vi "Lock to GPS.vi"(0 "niUsrpRio Session":T1={"FPGA Interface"=refnum, "RIO Interface Number"=0, "Data Clock Rate"=0, "FPGA Data Clock Rate"=0, "Global Settings Register Bus"=refnum, "Radio 0 Settings Register Bus"=refnum, "Radio 1 Settings Register Bus"=refnum, "Radio Settings Bus Semaphore"=refnum, "DB Queues"=[], "Characterization Data Valid?"=FALSE, "EEPROM Header"={"Checksum"=0, "Product Code"=0, "Hardware Current Version"=0, "Hardware Oldest Compatible Version"=0, "EEPROM Map Current Version"=0, "EEPROM Map Oldest Compatible Version"=0, "User Password"="", "Pointer to Factory Header"=0, "Pointer to User Header"=0, "Recommended Interval"=0, "Number of Reserved Bytes"=9, "Number of Daughterboards"=0, "Daughterboard IDs"=[], "Daughterboard Serial Numbers"=[]}, "Device Data Header"={"Checksum"=0, "Number of Channels"=0, "Number of Gain Settings"=[], "Pointer to Characterization Data"=[], "Number of Reserved Bytes"=27, "Number of Frequencies"=[]}, "EEPROM Characterization Header"={"Checksum"=0, "Date"=timestamp(0 s since 1904-01-01), "Temperature"=0.0, "Misc. Info"="", "Pointer to Device Data Header"=0, "Number of Reserved Bytes"=28}, "Characterization Data"=[], "FPGA Current Version"=0, "FPGA Oldest Compatible Version"=0, "Fixed Logic Current Version"=0, "Fixed Logic Oldest Compatible Version"=0, "FPGA Radio Settings Bus Current Version"=0, "FPGA Radio Settings Bus Oldest Compatible Version"=0, "FPGA Board Config Current Version"=0, "FPGA Board Config Oldest Compatible Version"=0, "Daughterboard Clock Rate"=0, "daughterboard configuration session handles"=[]} {"Daughterboard Clock Rate" format="%#.3pHz"; "FPGA Data Clock Rate" format="%#.3pHz"; "Data Clock Rate" format="%#.3pHz"; "Characterization Data"."Frequencies [Hz]" format="%#_6p"; "EEPROM Characterization Header"."Pointer to Device Data Header" format="%x"; "EEPROM Characterization Header"."Checksum" format="%x"; "Device Data Header"."Pointer to Characterization Data" format="%x"; "Device Data Header"."Checksum" format="%x"; "EEPROM Header"."Pointer to User Header" format="%x"; "EEPROM Header"."Pointer to Factory Header" format="%x"; "EEPROM Header"."Product Code" format="%x"; "EEPROM Header"."Checksum" format="%x"}, 1 "scope":string, 11 "error in":errorcluster) -> (4 "niUsrpRio Session (out)":T1={"FPGA Interface"=refnum, "RIO Interface Number"=0, "Data Clock Rate"=0, "FPGA Data Clock Rate"=0, "Global Settings Register Bus"=refnum, "Radio 0 Settings Register Bus"=refnum, "Radio 1 Settings Register Bus"=refnum, "Radio Settings Bus Semaphore"=refnum, "DB Queues"=[], "Characterization Data Valid?"=FALSE, "EEPROM Header"={"Checksum"=0, "Product Code"=0, "Hardware Current Version"=0, "Hardware Oldest Compatible Version"=0, "EEPROM Map Current Version"=0, "EEPROM Map Oldest Compatible Version"=0, "User Password"="", "Pointer to Factory Header"=0, "Pointer to User Header"=0, "Recommended Interval"=0, "Number of Reserved Bytes"=9, "Number of Daughterboards"=0, "Daughterboard IDs"=[], "Daughterboard Serial Numbers"=[]}, "Device Data Header"={"Checksum"=0, "Number of Channels"=0, "Number of Gain Settings"=[], "Pointer to Characterization Data"=[], "Number of Reserved Bytes"=27, "Number of Frequencies"=[]}, "EEPROM Characterization Header"={"Checksum"=0, "Date"=timestamp(0 s since 1904-01-01), "Temperature"=0.0, "Misc. Info"="", "Pointer to Device Data Header"=0, "Number of Reserved Bytes"=28}, "Characterization Data"=[], "FPGA Current Version"=0, "FPGA Oldest Compatible Version"=0, "Fixed Logic Current Version"=0, "Fixed Logic Oldest Compatible Version"=0, "FPGA Radio Settings Bus Current Version"=0, "FPGA Radio Settings Bus Oldest Compatible Version"=0, "FPGA Board Config Current Version"=0, "FPGA Board Config Oldest Compatible Version"=0, "Daughterboard Clock Rate"=0, "daughterboard configuration session handles"=[]} {"Daughterboard Clock Rate" format="%#.3pHz"; "FPGA Data Clock Rate" format="%#.3pHz"; "Data Clock Rate" format="%#.3pHz"; "Characterization Data"."Frequencies [Hz]" format="%#_6p"; "EEPROM Characterization Header"."Pointer to Device Data Header" format="%x"; "EEPROM Characterization Header"."Checksum" format="%x"; "Device Data Header"."Pointer to Characterization Data" format="%x"; "Device Data Header"."Checksum" format="%x"; "EEPROM Header"."Pointer to User Header" format="%x"; "EEPROM Header"."Pointer to Factory Header" format="%x"; "EEPROM Header"."Product Code" format="%x"; "EEPROM Header"."Checksum" format="%x"}, 15 "error out":errorcluster)   [LabVIEW 2020]
doc: "Locks to GPS. This VI blocks until the device locks to a GPS signal.\n\nThis VI will take between 10 seconds and 10 minutes to execute. The GPSDO requires 10 seconds at power on before polling for its lock status, and the GPSDO may take up to 10 minutes to acquire a GPS lock."
uses:
  <instrlib>/niUsrpRio/Config/v1/Host/Public/niUsrpRio Session.ctl
  <instrlib>/_niInstr/Register Bus/v0/Host/Public/Register Bus Session.ctl
  <instrlib>/_niInstr/Register Bus/v0/Host/Private/Session Data.ctl
  <instrlib>/niUsrpRio/Config/v1/Host/Private/DB Queue Reference.ctl
  <instrlib>/niUsrpRio/Config/v1/Host/Private/Daughterboard Data.ctl
  <instrlib>/niUsrpRio/Config/v1/Host/Private/ATR state data.ctl
  <instrlib>/niUsrpRio/Config/v1/Host/Private/Antenna Configuration.ctl
  <instrlib>/niUsrpRio/Config/v1/Host/Private/CPLD Power Mode.ctl
  <instrlib>/niUsrpRio/Config/v1/Host/Public/EEPROM Header.ctl
  <instrlib>/niUsrpRio/Config/v1/Host/Public/EEPROM Device Data Header.ctl
  <instrlib>/niUsrpRio/Config/v1/Host/Public/EEPROM Characterization Header.ctl
  <instrlib>/niUsrpRio/Config/v1/Host/Public/Characterization Data.ctl
  <instrlib>/niUsrpRio/Config/v1/Host/Public/IQ Imbalance.ctl
  <instrlib>/niUsrpRio/Config/v1/Host/Public/What to Wait for.ctl
  <instrlib>/niUsrpRio/Config/v1/Host/niUsrpRio Config v1 Host.lvlib
  <instrlib>/_niInstr/Register Bus/v0/Host/niInstr Register Bus v0 Host.lvlib
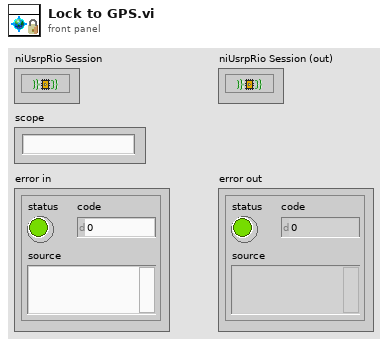
[diagram p1: front panel]
types:
  T1 = typedef "niUsrpRio Config v1 Host.lvlib/niUsrpRio Session.ctl" = cluster{"FPGA Interface":refnum<k20>, "RIO Interface Number":u32, "Data Clock Rate":u32, "FPGA Data Clock Rate":u32, "Global Settings Register Bus":T2, "Radio 0 Settings Register Bus":T2, "Radio 1 Settings Register Bus":T2, "Radio Settings Bus Semaphore":T3, "DB Queues":T4[], "Characterization Data Valid?":bool, "EEPROM Header":T5, "Device Data Header":T6, "EEPROM Characterization Header":T7, "Characterization Data":T8[], "FPGA Current Version":u32, "FPGA Oldest Compatible Version":u32, "Fixed Logic Current Version":u32, "Fixed Logic Oldest Compatible Version":u32, "FPGA Radio Settings Bus Current Version":u32, "FPGA Radio Settings Bus Oldest Compatible Version":u32, "FPGA Board Config Current Version":u32, "FPGA Board Config Oldest Compatible Version":u32, "Daughterboard Clock Rate":u32, "daughterboard configuration session handles":u64[]}
  T2 = typedef "niInstr Register Bus v0 Host.lvlib/Register Bus Session.ctl" = refnum<queue>
  T3 = typedef "Semaphore RefNum" = refnum<k1>
  T4 = typedef "niUsrpRio Config v1 Host.lvlib/DB Queue Reference.ctl" = refnum<queue>
  T5 = typedef "niUsrpRio Config v1 Host.lvlib/EEPROM Header.ctl" = cluster{"Checksum":u32, "Product Code":u16, "Hardware Current Version":u16, "Hardware Oldest Compatible Version":u16, "EEPROM Map Current Version":u16, "EEPROM Map Oldest Compatible Version":u16, "User Password":string, "Pointer to Factory Header":u32, "Pointer to User Header":u32, "Recommended Interval":u16, "Number of Reserved Bytes":i32, "Number of Daughterboards":u8, "Daughterboard IDs":u16[], "Daughterboard Serial Numbers":string[]}
  T6 = typedef "niUsrpRio Config v1 Host.lvlib/EEPROM Device Data Header.ctl" = cluster{"Checksum":u32, "Number of Channels":u8, "Number of Gain Settings":u16[], "Pointer to Characterization Data":u32[], "Number of Reserved Bytes":i32, "Number of Frequencies":u16[]}
  T7 = typedef "niUsrpRio Config v1 Host.lvlib/EEPROM Characterization Header.ctl" = cluster{"Checksum":u32, "Date":timestamp, "Temperature":sgl, "Misc. Info":string, "Pointer to Device Data Header":u32, "Number of Reserved Bytes":i32}
  T8 = typedef "niUsrpRio Config v1 Host.lvlib/Characterization Data.ctl" = cluster{"Gains[dB]":dbl[], "Frequencies [Hz]":dbl[], "IQ Imbalance Table":T9[], "Measured Gains[dB]":dbl[][]}
  T9 = typedef "niUsrpRio Config v1 Host.lvlib/IQ Imbalance.ctl" = cluster{"Gain Imbalance [linear]":dbl, "Phase Imbalance [radians]":dbl, "Offset":cdb}
  T10 = typedef "niUsrpRio Config v1 Host.lvlib/What to Wait for.ctl" = enum16{"Global Settings SPI Ready", "Radio Clocks Valid", "ADC Clock PLL Locked", "Clock Chip Locked", "LO Locked", "GPS Locked", "DRAM Ready", "GPS NMEA Data Ready", "DAC PLL Locked", "DAC Sync Locked", "ADC Data Valid"}
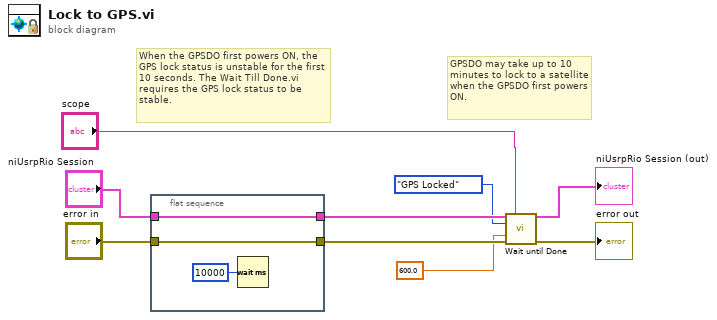
[diagram p0: block diagram]
diagram:
  # "GPSDO may take up to 10 minutes to lock to a satellite when the GPSDO first powers ON."
  # "When the GPSDO first powers ON, the GPS lock status is unstable for the first 10 seconds. The Wait Till Done.vi requires the GPS lock status to be stable."
  n1 = flat-sequence {
    tunnel: "niUsrpRio Session" -> [w11]
    tunnel: "error in" -> [w12]
    tunnel: [w12] -> w7
    tunnel: [w11] -> w6
    frame #0 {
      n2 = Wait (ms)(milliseconds to wait=u32 10000) -> ()  [unwired: 1 out]
    }
  }
  n3 = call <instrlib>:"Wait until Done.vi"("niUsrpRio Session"=w6, "scope"="scope", "What to Wait for"=What_to_Wait_for."GPS Locked", "timeout"=600.0 ("timeout (s)"), "error in"=w7) -> ("niUsrpRio Session (out)"=→"niUsrpRio Session (out)":T1, "error out"=→"error out":errorcluster)  [unwired: 9 in]
